vi "distributionPRofile.vi"(11 "prediction":sgl[][](array[numeric])) -> (2 "Array":dbl[][](array[numeric]))   [LabVIEW 2016]
uses:
  <vilib>/gmath/statdist.llb/Normal PDF.vi
  <vilib>/gmath/NI_Gmath.lvlib
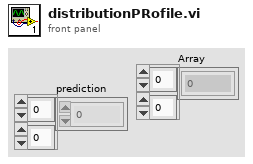
[diagram p1: front panel]
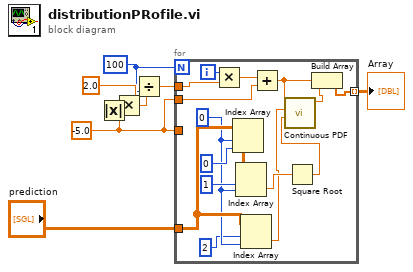
[diagram p0: block diagram]
diagram:
  w4 = 100
  w2 = -5.0
  n1 = Absolute Value(x=w2) -> (abs(x)=w7:dbl)
  n2 = Multiply(x=2.0, y=w7) -> (x*y=w5:dbl)
  n3 = Divide(x=w5, y=w4) -> (x/y=w3:dbl)
  n4 = for {
    N: w4 -> [_]
    tunnel: "prediction" -> [w21]
    tunnel: w2 -> [_]
    tunnel: w3 -> [w14]
    tunnel: w2 -> [w13]
    tunnel: [w11] -> w1 mode=indexing
    i -> [w15]
    w20 = 0 ("index (row)")
    n5 = Multiply(x=w15, y=w14) -> (x*y=w12:dbl)
    n6 = Index Array(array=w21, index (row)=w20, index (col)=0 ("index (row)")) -> ()  [unwired: 1 out]
    n7 = Index Array(array=w21, index (row)=1, index (col)=w20) -> (element=w18:sgl)
    n8 = Index Array(array=w21, index (row)=2, index (col)=w20) -> (element=w16:sgl)
    n9 = Add(x=w12, y=w13) -> (x+y=w9:dbl)
    n10 = Square Root(x=w18) -> (sqrt(x)=w17:sgl)
    n11 = call-poly <vilib>:"Continuous PDF.vi"("std"=w17, "mean"=w16, "x"=w9) -> ("pdf(x)"=w10:dbl)  [unwired: 7 in, 1 out]
    n12 = Build Array(w9, w10) -> (w11:dbl[])
  }
  "Array" <- w1
